vi "ziGetEventTreeChange.vi"(8 "Error In":errorcluster, 10 "TreeChange In":T1={"Timestamp (ticks)"=2149, "Action"=enum."Remove", "Name"=""}, 11 "Handle In":T2 {"Handle" format="0x%08x"; "Conn" format="0x%08x"}) -> (0 "Error Out":errorcluster, 2 "TreeChange Out":T1={"Timestamp (ticks)"=2149, "Action"=enum."Remove", "Name"=""}, 3 "Handle Out":T2 {"Handle" format="0x%08x"; "Conn" format="0x%08x"})   [LabVIEW 2019, in "Zurich Instruments LabOne.lvlib"]
uses:
  Zurich Instruments LabOne.lvlib
  ziTypeHandle.ctl
  ziTypeTreeChange.ctl
  Private/ziLV64.dll
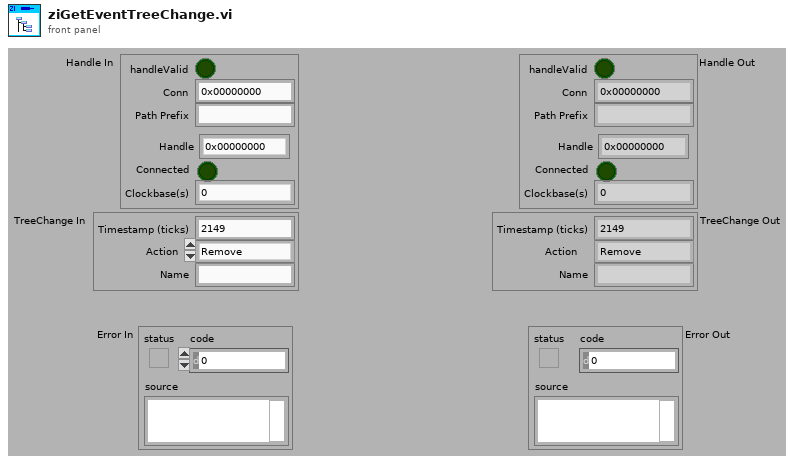
[diagram p1: front panel]
types:
  T1 = typedef "Zurich Instruments LabOne.lvlib/ziTypeTreeChange.ctl" = cluster{"Timestamp (ticks)":u64, "Action":enum32{"Remove", "Add", "Change"}, "Name":string}
  T2 = typedef "Zurich Instruments LabOne.lvlib/ziTypeHandle.ctl" = cluster{"handleValid":bool, "Conn":u64, "Path Prefix":string, "Handle":u64, "Connected":bool, "Clockbase(s)":dbl}
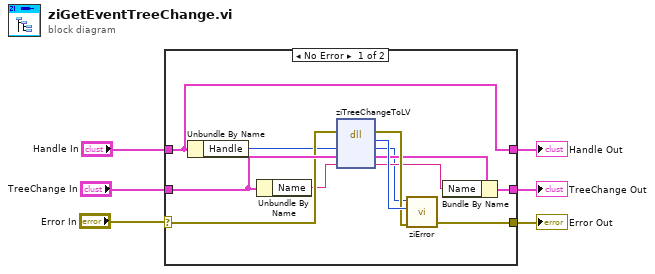
[diagram p0: block diagram]
diagram:
  n1 = case shown="No Error" "Error In" {
    selector: "Error In" -> [w15 w21]
    tunnel: "TreeChange In" -> [w18 w20]
    tunnel: [w17 w20] -> w5
    tunnel: [w16 w21] -> w4
    tunnel: [w8 w19] -> w3
    tunnel: "Handle In" -> [w8 w19]
    frame No Error {
      n2 = Unbundle By Name(w8) -> ("Handle"=w13:u64)
      n3 = Unbundle By Name(w18) -> ("Name"=w11:string)
      n4 = dll-call lib="G:/01_software/CryoTUM/sub_vi-s/Equipment/Zurich Instruments LabOne/Private/ziLV*.*" fn="ziTreeChangeToLV"(error in=w15, "ziEventBuffer"=w13, "TreeChangeCluster"=w18, "name"=w11) -> (error out=w12:errorcluster, "return type"=w14:u32, "ziEventBuffer"=w7:u64, "TreeChangeCluster"=w9:T1, "name"=w10:string)  [unwired: 2 in, 1 out]
      n5 = call "ziError.vi"("Conn"=w7, "ziErrorCode"=w14, "Error In"=w12) -> ("Error Out"=w16:errorcluster)  [unwired: 2 in, 1 out]
      n6 = Bundle By Name(cluster=w9, "Name"=w10) -> (w17:T1)
    }
    frame Error {
    }
  }
  "Handle Out" <- w3
  "TreeChange Out" <- w5
  "Error Out" <- w4
